vi "Set Main FPGA Chassis Slots Programming Mode.vi"(8 "error in (no error)":errorcluster, 10 "serverName in":string="10.0.18.244", 11 "Item Ref in":T1 format="%.0x") -> (0 "error out":errorcluster, 2 "serverName out":string="10.0.18.244", 3 "Item Ref out":T1 format="%.0x")   [LabVIEW 2017, in "Scan Engine Custom Device.lvlib"]
doc: "Goal of this VI is to set the slot \"Programming Mode\" property for recent cRIO chassis (NI-904x, NI-905x,...) in accordance to control \"FPGA / Scan interface mode\" control of Target main Configuration page, in \"Othe Settings\" section.\n------------------------------------------------------------------------------------------------------\nIMPLEMENTATION\nThis VI checks the value of property \"FPGA / Scan interface mode\" of Target Configuration Page."
uses:
  <vilib>/NI Veristand/Custom Device API/Custom Device Item Ref.ctl
  Type Defs/FPGAScanInterfaceMode.ctl
  NationalInstruments.VeriStand.SystemDefinitionAPI
  Scan Engine Custom Device.lvlib
  <vilib>/NI Veristand/Custom Device Tools/Custom Device Utility Library/Custom Device Utility Library.lvlib
  <vilib>/NI Veristand/Custom Device Offline API/Custom Device Offline API.lvlib
  <vilib>/NI Veristand/Custom Device API/Custom Device API.lvlib
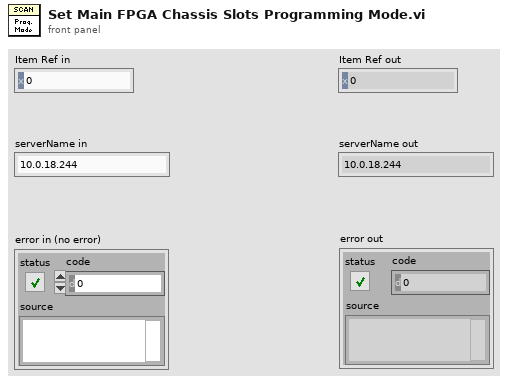
[diagram p1: front panel]
types:
  T1 = typedef "Custom Device API.lvlib/Custom Device Item Ref.ctl" = u64
  T2 = typedef "Scan Engine Custom Device.lvlib/FPGAScanInterfaceMode.ctl" = enum16{"Use Current", "FPGA", "Scan mode"}
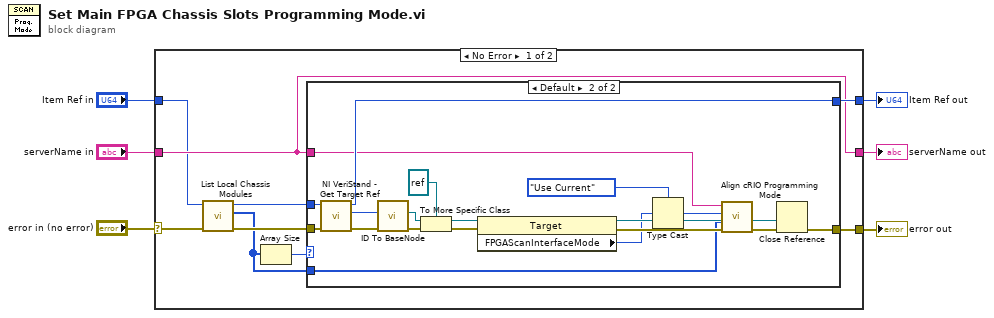
[diagram p0: block diagram]
diagram:
  n1 = case shown="No Error" "error in (no error)" {
    selector: "error in (no error)" -> [w11 w39]
    tunnel: [w14 w39] -> w5
    tunnel: "Item Ref in" -> [w12 w38]
    tunnel: [w15 w38] -> w3
    tunnel: "serverName in" -> [w13 w37]
    tunnel: [w13 w37] -> w1
    frame No Error {
      n2 = call "List Local Chassis Modules.vi"("error in (no error)"=w11, "Item Ref in"=w12) -> ("error out"=w9:errorcluster, "Local Slots #"=w7:u32[], "Item Ref out"=w10:T1)  [unwired: 7 in]
      n3 = Array Size(array=w7) -> (size(s)=w8:i32)
      n4 = case shown="Default" w8 {
        tunnel: [w17 w32] -> w15
        tunnel: [w16 w28] -> w14
        tunnel: w13 -> [_ w25]
        tunnel: w10 -> [w17 w22]
        tunnel: w9 -> [w16 w21]
        tunnel: w7 -> [_ w20]
        frame 0 {
          # "No modules configured in Local Chassis in Sysdef."
        }
        frame Default {
          n5 = call <vilib>:"NI VeriStand - Get Target Ref.vi"("error in"=w21, "Item Ref in"=w22) -> ("error out"=w31:errorcluster, "Target Ref"=w36:T1, "Item Ref out"=w32:T1)  [unwired: 6 in, 1 out]
          n6 = call <vilib>:"ID To BaseNode.vi"("error in (no error)"=w31, "ID in"=w36) -> ("error out"=w30:errorcluster, "BaseNode"=w34:refnum<k24>)  [unwired: 7 in, 1 out]
          n7 = To More Specific Class(target class=refnum<k24> refnum, reference=w34, error in=w30) -> (specific class reference=w35:refnum<k24>, error out=w29:errorcluster)
          n8 = property class="Target"(reference=w35, error in=w29) -> (reference out=w27:refnum<k24>, error out=w24:errorcluster, "FPGAScanInterfaceMode"=w19:u16)
          n9 = Type Cast(type=FPGAScanInterfaceMode."Use Current" ("Enum"), x=w19) -> (*(type *) &x=w23:T2)
          n10 = call "Align cRIO Programming Mode.vi"("error in (no error)"=w24, "Local Slots #"=w20, "FPGAScanInterfaceMode"=w23, "Target (localhost)"=w25) -> ("error out"=w26:errorcluster)  [unwired: 5 in, 2 out]
          n11 = Close Reference(reference=w27, error in (no error)=w26) -> (error out=w28:errorcluster)
        }
      }
    }
    frame Error {
    }
  }
  "error out" <- w5
  "Item Ref out" <- w3
  "serverName out" <- w1
